vi "SPECTRAL ANALYSIS.vi"() -> ()   [LabVIEW 2019]
uses:
  <vilib>/Analysis/2dsp.llb/Real FFT.vi
  <vilib>/Analysis/2dsp.llb/Inverse Real FFT.vi
  <vilib>/Analysis/2dsp.llb/Power Spectrum (DBL).vi
  <vilib>/Analysis/NI_AALPro.lvlib
  <vilib>/gmath/NI_Gmath.lvlib
panel:
  out "INVERSE FFT":dbl[](graph)
  out "LAPLACE":dbl[](graph)
  out "FFT":dbl[](graph)
  out "PSD":dbl[](graph)
  out "INPUT":dbl[](graph)
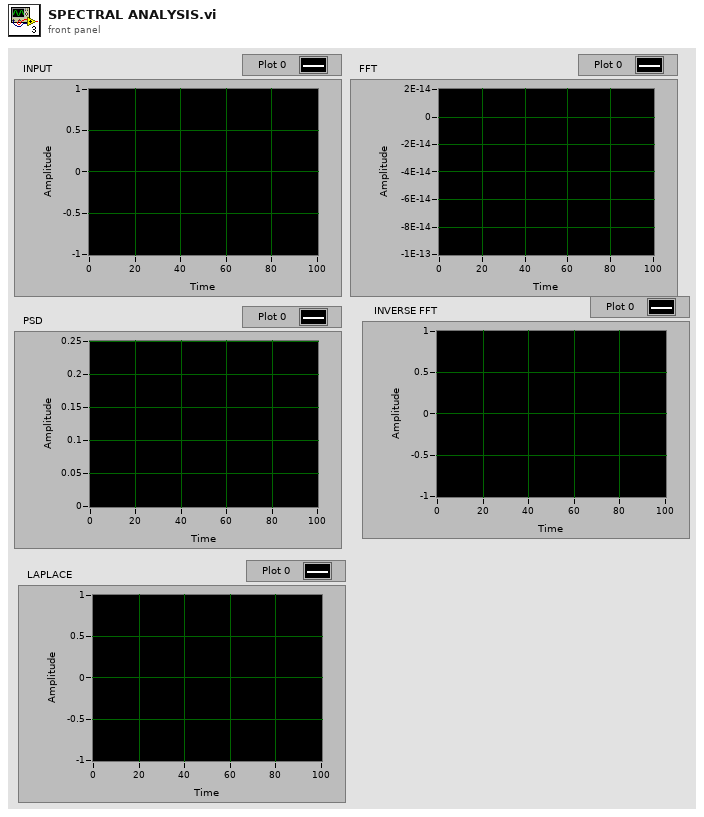
[diagram p1: front panel]
types:
  T1 = enum16{"sine", "cosine", "triangle", "square", "sawtooth", "increasing ramp", "decreasing ramp"}
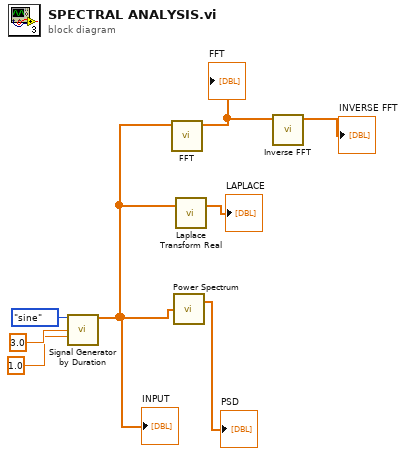
[diagram p0: block diagram]
diagram:
  n1 = call <vilib>:"Signal Generator by Duration.vi"("signal type"=T1."sine", "frequency"=3.0, "amplitude"=1.0) -> ("signal"=w4:dbl[])  [unwired: 9 in, 3 out]
  "INPUT" <- w4
  n2 = call-poly <vilib>:"FFT.vi"("X"=w4) -> ("FFT {X}"=w2:cdb[])  [unwired: 9 in, 1 out]
  "FFT" <- w2
  n3 = call-poly <vilib>:"Power Spectrum.vi"("X"=w4) -> ("Power Spectrum"=→"PSD":dbl[])  [unwired: 1 out]
  n4 = call <vilib>:"Laplace Transform Real.vi"("X"=w4) -> ("Laplace {X}"=→"LAPLACE":dbl[])  [unwired: 1 in, 1 out]
  n5 = call-poly <vilib>:"Inverse FFT.vi"("FFT {X}"=w2) -> ("X"=→"INVERSE FFT":dbl[])  [unwired: 9 in, 1 out]
